vi "ManipWaitForDrive.vi"(3 "Parameter String":string) -> (0 "Error Out":errorcluster, 1 "Advance Trigger":bool)   [LabVIEW 2023]
doc: "This VI pauses the manipulator sequencer until the drive sequencer has reached (or passed) the specified step.\n\nParameters:\nParam1: manipulator step to wait for"
uses:
  SafeParser_Integer.vi
  GlobalAutonomous.vi
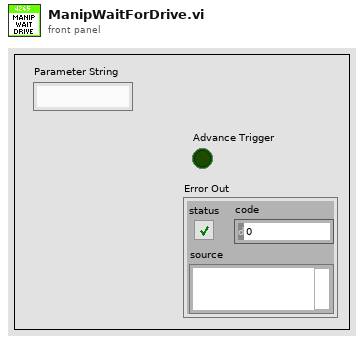
[diagram p1: front panel]
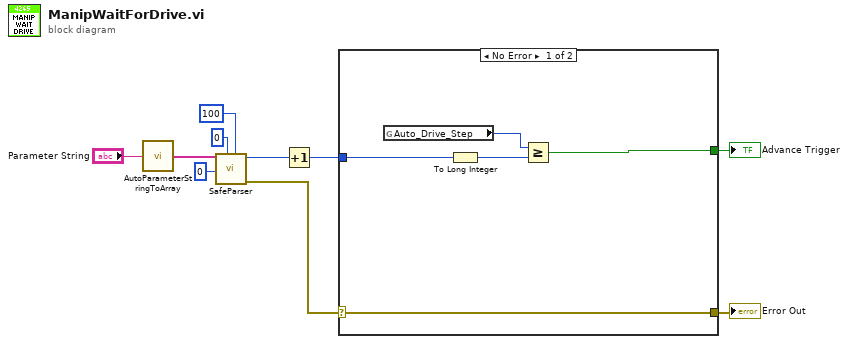
[diagram p0: block diagram]
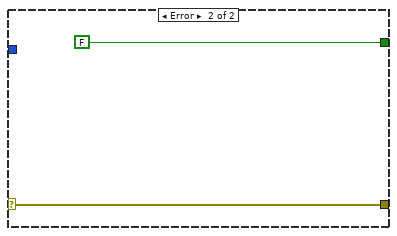
[diagram p2: hidden frame]
diagram:
  n1 = call "AutoParameterStringToArray.vi"("Parameter String"="Parameter String") -> ("Parsed Parameters"=w3:string[])
  n2 = call-poly "SafeParser.vi"("Maximum"=100, "Minimum"=0, "Array Index"=0 ("Parameter Index"), "String Array"=w3) -> ("Error Out"=w2:errorcluster, "Typecast  Value"=w7:i32)  [unwired: 6 in]
  n3 = Increment(x=w7) -> (x+1=w1:i32)
  n4 = case shown="No Error" w2 {
    selector: w2 -> [w15 w17]
    tunnel: [w11 FALSE] -> w10
    tunnel: [w15 w17] -> w9
    tunnel: w1 -> [w12 _]
    frame No Error {
      n5 = global read "GlobalAutonomous.vi" "Auto_Drive_Step"() -> (w14:i32)
      n6 = To Long Integer(number=w12) -> (32bit integer=w13:i32)
      n7 = Greater Or Equal?(x=w14, y=w13) -> (x >= y?=w11:bool)
    }
    frame Error {
    }
  }
  "Advance Trigger" <- w10
  "Error Out" <- w9
